vi "MakeLegend.vi"(11 "NavigationsDetails":cluster{T2[]}[](array[cluster])) -> (1 "Uniques":T1, 3 "PlantUMLText":string)   [LabVIEW 2021, in "ButtonBarFlow.lvlib"]
uses:
  ButtonBarFlow.lvlib
  ActiveObjects/VerticalButtonBar/ButtonCollection/ButtonDefinition.ctl
  469aed49-2bbe-4f3c-901e-33780b3043e4.vi
  48343e22-bfcc-4ed4-9558-109764ff3ad5.vi
  681623b6-0f21-4363-b3c0-82af1974f68a.vi
  732340fd-f00a-433b-b7d5-f815e438fdb2.vi
  3e8ce2a2-6066-459b-91af-94707ddede46.vi
  ActiveObjects/VerticalButtonBar/ButtonCollection/ButtonCollection.lvclass
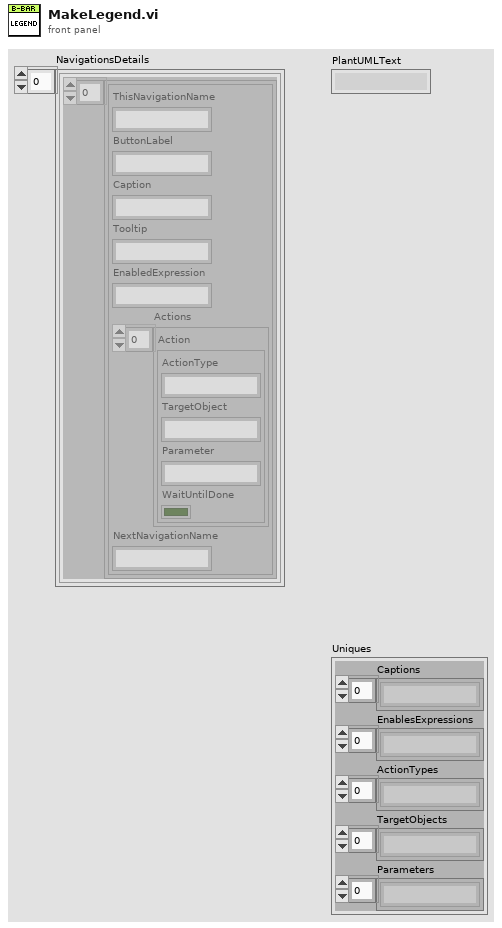
[diagram p1: front panel]
types:
  T1 = cluster{"Captions":string[], "EnablesExpressions":string[], "ActionTypes":string[], "TargetObjects":string[], "Parameters":string[]}
  T2 = typedef "ButtonCollection.lvclass/ButtonDefinition.ctl" = cluster{"ThisNavigationName":string, "ButtonLabel":string, "Caption":string, "Tooltip":string, "EnabledExpression":string, "Actions":cluster{"ActionType":string, "TargetObject":string, "Parameter":string, "WaitUntilDone":bool}[], "NextNavigationName":string}
  T3 = cluster{"ActionType":string, "TargetObject":string, "Parameter":string, "WaitUntilDone":bool}[]
  T4 = cluster{"array with duplicates removed":string[], "array with duplicates removed":string[], "array with duplicates removed":string[], "array with duplicates removed":string[], "array with duplicates removed":string[]}
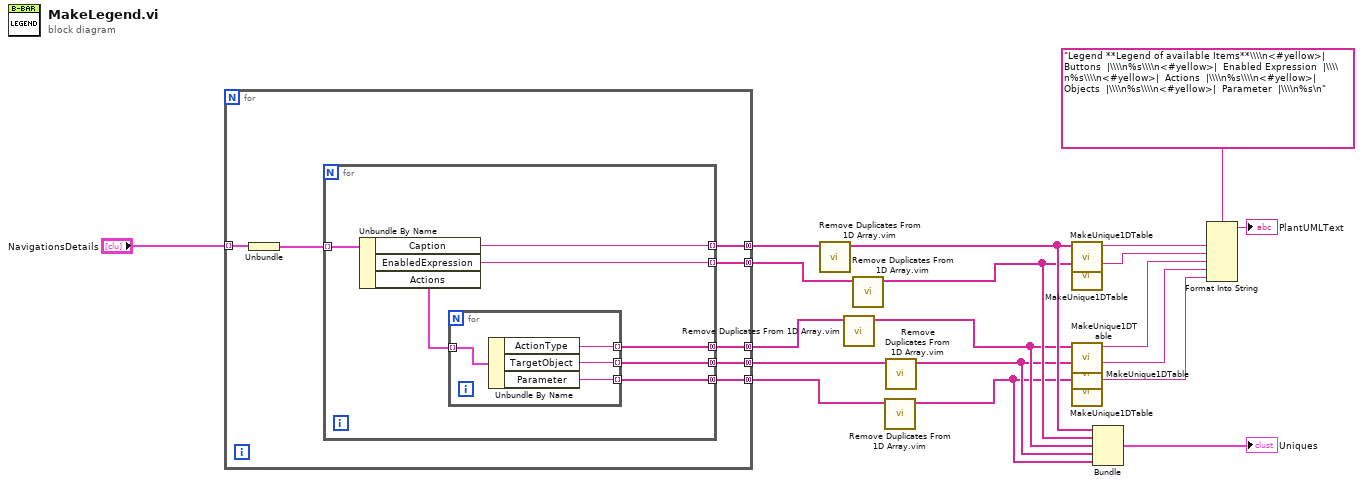
[diagram p0: block diagram]
diagram:
  n1 = for {
    tunnel: "NavigationsDetails" -> [w26] mode=indexing
    tunnel: [w24] -> w17 mode=concatenating
    tunnel: [w23] -> w11 mode=concatenating
    tunnel: [w22] -> w10 mode=concatenating
    tunnel: [w21] -> w19 mode=concatenating
    tunnel: [w20] -> w12 mode=concatenating
    n2 = Unbundle(w26) -> (w25:T2[])
    n3 = for {
      tunnel: w25 -> [w33] mode=indexing
      tunnel: [w31] -> w24 mode=concatenating
      tunnel: [w30] -> w23 mode=concatenating
      tunnel: [w29] -> w22 mode=concatenating
      tunnel: [w28] -> w21 mode=indexing
      tunnel: [w27] -> w20 mode=indexing
      n4 = Unbundle By Name(w33) -> ("Caption"=w28:string, "EnabledExpression"=w27:string, "Actions"=w32:T3)
      n5 = for {
        tunnel: w32 -> [w37] mode=indexing
        tunnel: [w36] -> w31 mode=indexing
        tunnel: [w35] -> w30 mode=indexing
        tunnel: [w34] -> w29 mode=indexing
        n6 = Unbundle By Name(w37) -> ("ActionType"=w36:string, "TargetObject"=w35:string, "Parameter"=w34:string)
      }
    }
  }
  n7 = call "Remove Duplicates From 1D Array.vim"("array"=w19) -> ("array with duplicates removed"=w6:string[])  [unwired: 10 in]
  n8 = call "Remove Duplicates From 1D Array.vim"("array"=w17) -> ("array with duplicates removed"=w4:string[])  [unwired: 10 in]
  n9 = call "Remove Duplicates From 1D Array.vim"("array"=w12) -> ("array with duplicates removed"=w5:string[])  [unwired: 10 in]
  n10 = call "Remove Duplicates From 1D Array.vim"("array"=w10) -> ("array with duplicates removed"=w2:string[])  [unwired: 10 in]
  n11 = call "Remove Duplicates From 1D Array.vim"("array"=w11) -> ("array with duplicates removed"=w3:string[])  [unwired: 10 in]
  n12 = call "MakeUnique1DTable.vi"("Array"=w6) -> ("String"=w8:string)  [unwired: 10 in]
  n13 = call "MakeUnique1DTable.vi"("Array"=w5) -> ("String"=w9:string)  [unwired: 10 in]
  n14 = call "MakeUnique1DTable.vi"("Array"=w4) -> ("String"=w16:string)  [unwired: 10 in]
  n15 = call "MakeUnique1DTable.vi"("Array"=w3) -> ("String"=w15:string)  [unwired: 10 in]
  n16 = call "MakeUnique1DTable.vi"("Array"=w2) -> ("String"=w14:string)  [unwired: 10 in]
  n17 = Bundle("array with duplicates removed"=w6, "array with duplicates removed"=w5, "array with duplicates removed"=w4, "array with duplicates removed"=w3, "array with duplicates removed"=w2) -> (→"Uniques":T4)  [unwired: 1 in]
  n18 = Format Into String(format string="Legend **Legend of available Items**\\\\n<#yellow>|  Buttons  |\\\\n%s\\\\n<#yellow>|  Enabled Expression  |\\\\n%s\\\\n<#yellow>|  Actions  |\\\\n%s\\\\n<#yellow>|  Objects  |\\\\n%s\\\\n<#yellow>|  Parameter  |\\\\n%s\n", w8, w9, w16, w15, w14) -> (resulting string=→"PlantUMLText":string)  [unwired: 2 in, 1 out]
